vi "_1Hello_World.vi"() -> ()   [LabVIEW 2018]
panel:
  out "String":string
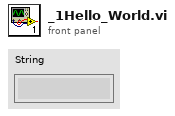
[diagram p1: front panel]
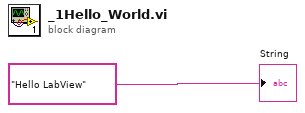
[diagram p0: block diagram]
diagram:
  "String" <- "Hello LabView"
